vi "Butterfly_PullUp Capacitance.vi"(0 "Semiconductor Module Context":T2, 1 "SMU_PD_PU_5V_pin":string[](array[string])=["VDD"], 2 "SMU_PD_PU_5v_v":dbl=5.0 format="%_6p", 3 "C_TH_Delta":dbl=0.03 format="%#_13g", 4 "VNAs Measurement Parameters":T1, 5 "error in (no error)":errorcluster, 9 "Start_v":dbl=10.0 format="%#_13g", 11 "Stop_v":dbl=41.0 format="%#_13g") -> (14 "Semiconductor Module Context Out":T2, 19 "error out":errorcluster)   [LabVIEW 2013]
uses:
  <vilib>/NI_TestStand_SemiconductorModule/NI_TestStand_Semiconductor_Module.lvlibp/PinMap/General/SemiconductorModuleContext.ctl
  VNA/VNAs Measurement Parameters.ctl
  <instrlib>/niDCPower/nidcpower.llb/niDCPower Wait For Event - Event.ctl
  <vilib>/NI_TestStand_SemiconductorModule/NI_TestStand_Semiconductor_Module.lvlibp/PinMap/DC Power/PinToNIDCPowerSession.vi
  <vilib>/NI_TestStand_SemiconductorModule/NI_TestStand_Semiconductor_Module.lvlibp/PinMap/General/Publish/PublishDataDouble2D.vi
  <vilib>/NI_TestStand_SemiconductorModule/NI_TestStand_Semiconductor_Module.lvlibp
  VNA/Pin Map API/VNA Custom Instrument.lvlib
panel:
  in  "PD_Pin":string="SMU_PD"
  out "Site":i32
  out "RL Step":i32
  out "PI Step":i32
  out "C_TH_PU":dbl format="%#_3g"
  out "C_Free":dbl[](array[numeric]) format="%#_3g"
  out "max index":i32
  out "BF C PI":dbl format="%#_3g"
  out "C_VPI":dbl
  out "BF C RL":dbl format="%#_3g"
  out "C_VRL":dbl
  out "appended array":dbl[][](array[numeric]) format="%#_3g"
  out "S3 steps":dbl[](array[numeric]) format="%#_3g"
  out "S2 steps":dbl[](array[numeric]) format="%#_3g"
  out "S1 steps":dbl[](array[numeric]) format="%#_3g"
  out "S0 steps":dbl[](array[numeric]) format="%#_3g"
  out "BF values":dbl[](array[numeric])
  out "VRLs":dbl[](array[numeric])
  out "VPIs":dbl[](array[numeric])
  out "Multisite Cap Data":dbl[][][](array[numeric])
  out "BF Names":string[](array[string])
  out "BFSamples":i32
  in  "Step_v":dbl=1.0
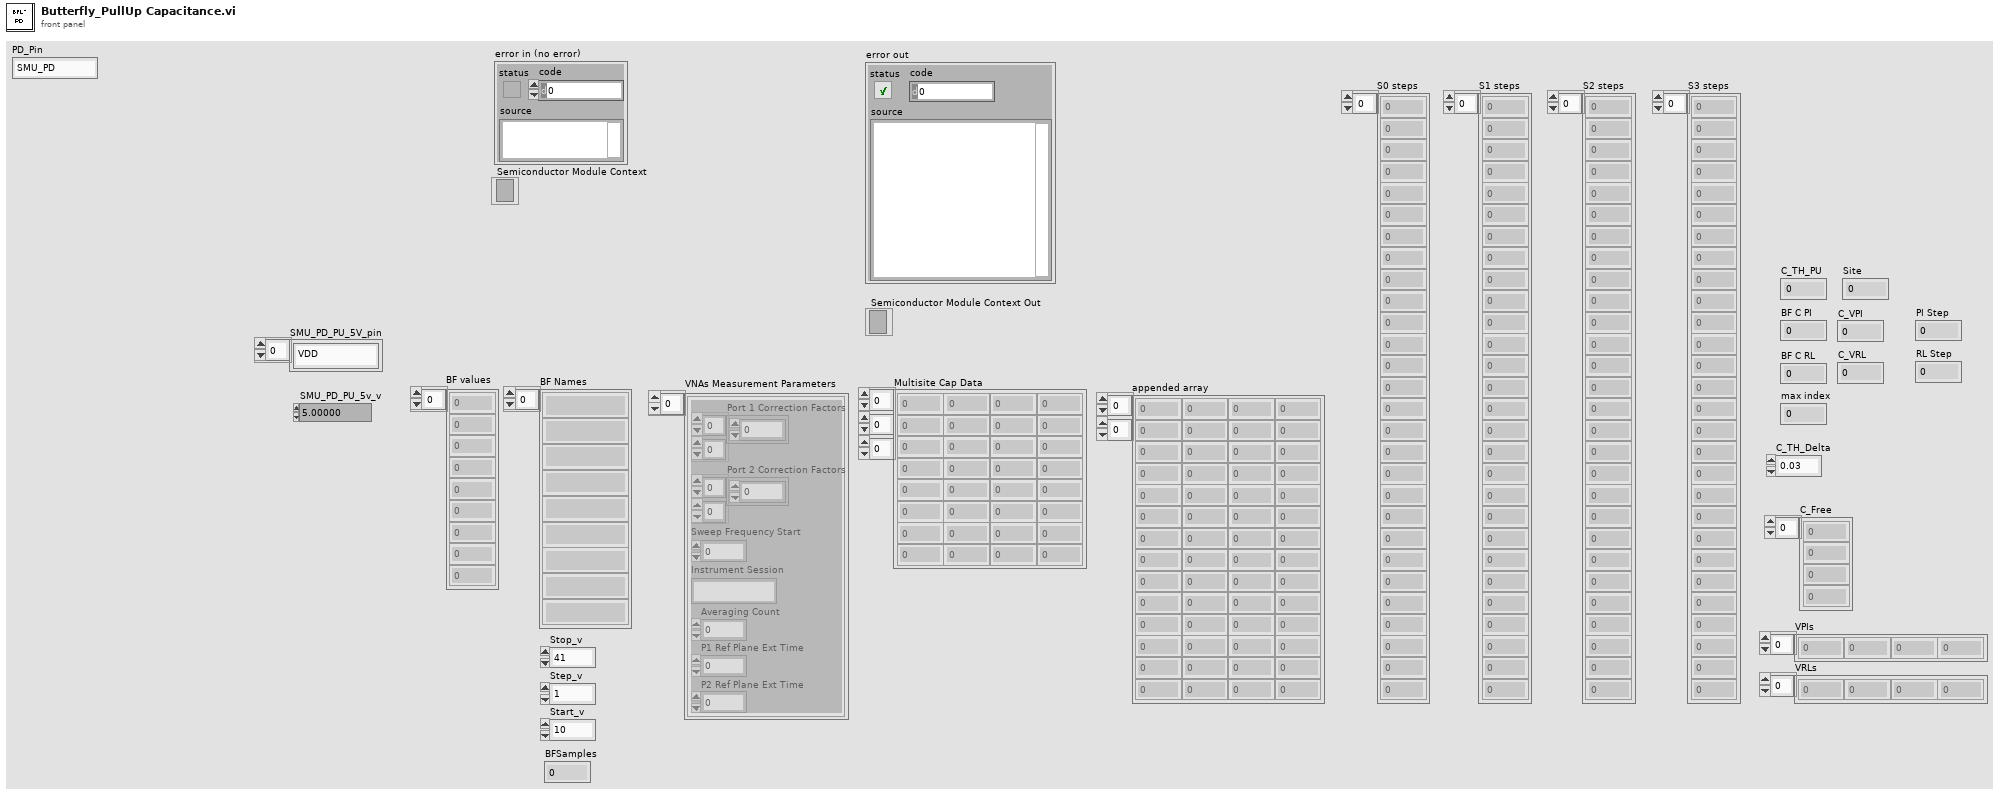
[diagram p1: front panel]
types:
  T1 = typedef "VNAs Measurement Parameters.ctl" = cluster{"Port 1 Correction Factors":cdb[][], "Port 2 Correction Factors":cdb[][], "Sweep Frequency Start":dbl, "Instrument Session":string, "Averaging Count":i32, "P1 Ref Plane Ext Time":dbl, "P2 Ref Plane Ext Time":dbl}[]
  T2 = typedef "NI_TestStand_Semiconductor_Module.lvlibp/SemiconductorModuleContext.ctl" = refnum<k7>
  T3 = typedef "niDCPower Wait For Event - Event.ctl" = i32
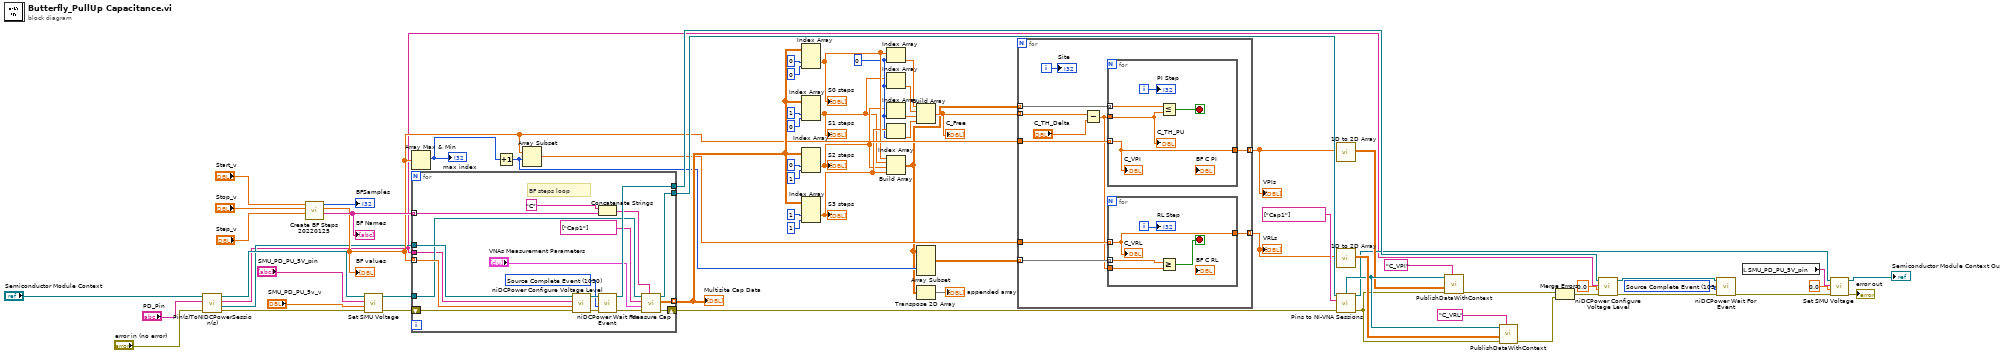
[diagram p0: block diagram]
diagram:
  w25 = 0 ("index")
  w57 = T3 1030 items=["Source Complete Event"=1030, "Measure Complete Event"=1031, "Sequence Iteration Complete Event"=1032, "Sequence Engine Done Event"=1033, "Pulse Complete Event"=1051, "Ready For Pulse Trigger Event"=1052] ("event")
  n1 = call-poly <vilib>:"Pin(s)ToNIDCPowerSession(s).vi"("error in (no error)"="error in (no error)", "Pin"="PD_Pin", "Semiconductor Module Context"="Semiconductor Module Context") -> ("error out"=w2:errorcluster, "Instrument Session"=w4:refnum<k15>, "Channel List"=w1:string, "Semiconductor Module Context Out"=w5:T2)  [unwired: 4 in, 1 out]
  n2 = call "Create BF Steps 20220125.vi"("Step_v"="Step_v", "Stop_v"="Stop_v", "Start_v"="Start_v") -> ("BF Names"=w62:string[], "BF values"=w32:dbl[], "BFSamples"=→"BFSamples":i32)  [unwired: 6 in]
  "BF Names" <- w62
  "BF values" <- w32
  n3 = call "Set SMU Voltage.vi"("error in (no error)"=w2, "VDD voltage level"="SMU_PD_PU_5v_v", "Pins"="SMU_PD_PU_5V_pin", "Semiconductor Module Context"=w5) -> ("error out"=w17:errorcluster, "Semiconductor Module Context Out"=w14:T2)  [unwired: 5 in, 1 out]
  n4 = Array Max & Min(array=w32) -> (max index (indices)=w34:i32)  [unwired: 3 out]
  "max index" <- w34
  n5 = for {
    shift-right: [w75] -> w55
    shift-left: w17 -> [w80]
    tunnel: w14 -> [w73]
    tunnel: [w72] -> w67
    tunnel: [w71] -> w56 mode=indexing
    tunnel: w62 -> [w84] mode=indexing
    tunnel: w32 -> [w79] mode=indexing
    tunnel: w4 -> [w78]
    tunnel: [w77] -> w60
    tunnel: w1 -> [w69]
    w82 = T3 1030 items=["Source Complete Event"=1030, "Measure Complete Event"=1031, "Sequence Iteration Complete Event"=1032, "Sequence Engine Done Event"=1033, "Pulse Complete Event"=1051, "Ready For Pulse Trigger Event"=1052] ("event")
    # "BF steps loop"
    n6 = call <instrlib>:"niDCPower Configure Voltage Level.vi"("error in (no error)"=w80, "voltage level"=w79, "channel name"=w69, "instrument handle"=w78) -> ("error out"=w81:errorcluster, "instrument handle out"=w83:refnum<k15>)  [unwired: 6 in]
    n7 = Concatenate Strings("C" ("string"), w84) -> (w74:string)
    n8 = call <instrlib>:"niDCPower Wait For Event.vi"("error in (no error)"=w81, "event"=w82, "instrument handle"=w83) -> ("error out"=w76:errorcluster, "instrument handle out"=w77:refnum<k15>)  [unwired: 7 in]
    n9 = call "Measure Cap.vi"("Measurement Id"=w74, "error in (no error)"=w76, "VNAs Measurement Parameters"="VNAs Measurement Parameters", "Pins"=string[] ["Cap1"] ("Capacitance Pins"), "Semiconductor Module Context"=w73) -> ("error out"=w75:errorcluster, "Multisite Cap Data"=w71:dbl[][], "Semiconductor Module Context Out"=w72:T2)  [unwired: 4 in]
  }
  "Multisite Cap Data" <- w56
  n10 = Increment(x=w34) -> (x+1=w33:i32)
  n11 = Array Subset(array=w32, index=w33) -> (w31:dbl[])  [unwired: 1 in]
  n12 = Index Array(array=w56, index (dim 1)=0 ("disabled index (row)"), index (dim 2)=0 ("disabled index (col)")) -> (element=w28:dbl[])  [unwired: 1 in]
  "S0 steps" <- w28
  n13 = Index Array(array=w56, index (dim 1)=1 ("index (row)"), index (dim 2)=0 ("index (col)")) -> (element=w19:dbl[])  [unwired: 1 in]
  "S1 steps" <- w19
  n14 = Index Array(array=w56, index (dim 1)=0 ("index (row)"), index (dim 2)=1 ("index (col)")) -> (element=w20:dbl[])  [unwired: 1 in]
  "S2 steps" <- w20
  n15 = Index Array(array=w56, index (dim 1)=1 ("index (row)"), index (dim 2)=1 ("index (col)")) -> (element=w26:dbl[])  [unwired: 1 in]
  "S3 steps" <- w26
  n16 = Index Array(array=w28, index=w25) -> (element=w27:dbl)
  n17 = Index Array(array=w19, index=w25) -> (element=w24:dbl)
  n18 = Index Array(array=w20, index=w25) -> (element=w22:dbl)
  n19 = Index Array(array=w26, index=w25) -> (element=w23:dbl)
  n20 = Build Array(w28, w19, w20, w26) -> (w18:dbl[][])
  n21 = Build Array(w27, w24, w22, w23) -> (w21:dbl[])
  "C_Free" <- w21
  n22 = Array Subset(array=w18, index (col)=w33) -> (w35:dbl[][])  [unwired: 3 in]
  n23 = Transpose 2D Array(2D array=w18) -> (transposed array=→"appended array":dbl[][])
  n24 = for {
    tunnel: w32 -> [w95]
    tunnel: [w94] -> w30 mode=indexing
    tunnel: w31 -> [w93]
    tunnel: w35 -> [w92] mode=indexing
    tunnel: [w91] -> w29 mode=indexing
    tunnel: w21 -> [w88] mode=indexing
    tunnel: w18 -> [w89] mode=indexing
    i -> [w90]
    n25 = Subtract(x=w88, y="C_TH_Delta") -> (x-y=w86:dbl)
    n26 = for {
      tunnel: w95 -> [w104] mode=indexing
      tunnel: [w104] -> w94
      tunnel: w86 -> [w103]
      tunnel: w89 -> [w101] mode=indexing
      i -> [w102]
      stop <- w105 stop-if-true
      n27 = Less Or Equal?(x=w101, y=w103) -> (x <= y?=w105:bool)
      "C_VPI" <- w104
      "C_TH_PU" <- w103
      "PI Step" <- w102
    }
    n28 = for {
      tunnel: w93 -> [w99] mode=indexing
      tunnel: w92 -> [w96] mode=indexing
      tunnel: [w99] -> w91
      tunnel: w86 -> [w98]
      i -> [w97]
      stop <- w100 stop-if-true
      n29 = Greater Or Equal?(x=w96, y=w98) -> (x >= y?=w100:bool)
      "C_VRL" <- w99
      "RL Step" <- w97
    }
    "Site" <- w90
  }
  "VPIs" <- w30
  "VRLs" <- w29
  n30 = call "1D to 2D Array.vi"("1D Array"=w30) -> ("2D Array"=w39:dbl[][])  [unwired: 10 in]
  n31 = call "1D to 2D Array.vi"("1D Array"=w29) -> ("2D Array"=w52:dbl[][])  [unwired: 10 in]
  n32 = call "Pins to NI-VNA Sessions.vi"("Semiconductor Module Context"=w67, "Pins"=string[] ["Cap1"] ("Capacitance Pins"), "error in (no error)"=w55) -> ("Pin Query Context"=w40:refnum<class "MultiplePinMultipleSessionQueryContext.lvclass">, "Semiconductor Module Context Out"=w12:T2, "error out"=w36:errorcluster)  [unwired: 8 in, 2 out]
  n33 = call-poly <vilib>:"PublishDataWithContext.vi"("Published Data Id"="C_VPI", "error in (no error)"=w36, "Data In"=w39, "Pin Query Context"=w40) -> ("error out"=w37:errorcluster)  [unwired: 6 in, 1 out]
  n34 = call-poly <vilib>:"PublishDataWithContext.vi"("Published Data Id"="C_VRL", "error in (no error)"=w36, "Data In"=w52, "Pin Query Context"=w40) -> ("error out"=w53:errorcluster)  [unwired: 6 in, 1 out]
  n35 = Merge Errors(w37, w53) -> (w54:errorcluster)
  n36 = call <instrlib>:"niDCPower Configure Voltage Level.vi"("error in (no error)"=w54, "voltage level"=0.0, "channel name"=w1, "instrument handle"=w60) -> ("error out"=w59:errorcluster, "instrument handle out"=w58:refnum<k15>)  [unwired: 6 in]
  n37 = call <instrlib>:"niDCPower Wait For Event.vi"("error in (no error)"=w59, "event"=w57, "instrument handle"=w58) -> ("error out"=w15:errorcluster)  [unwired: 7 in, 1 out]
  n38 = local read "SMU_PD_PU_5V_pin"() -> (w10:string[])
  n39 = call "Set SMU Voltage.vi"("error in (no error)"=w15, "VDD voltage level"=0.0, "Pins"=w10, "Semiconductor Module Context"=w12) -> ("error out"=→"error out":errorcluster, "Semiconductor Module Context Out"=→"Semiconductor Module Context Out":T2)  [unwired: 5 in, 1 out]
